vi "Autosort Get Sort Option.vi"(11 "Index":i32) -> (3 "Autosort Parameters":T1)   [LabVIEW 2016]
uses:
  Autosort Parameters.ctl
  Autosort Parameters Set.vi
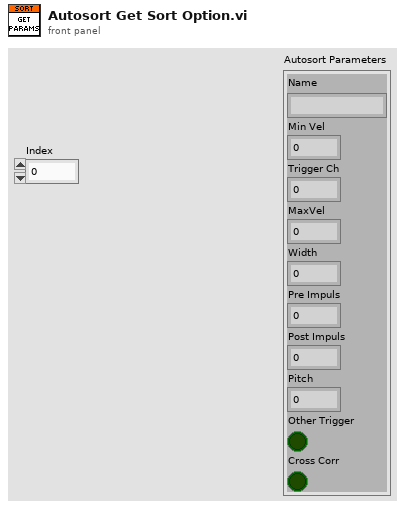
[diagram p1: front panel]
types:
  T1 = typedef "Autosort Parameters.ctl" = cluster{"Name":string, "Min Vel":dbl, "Trigger Ch":i32, "MaxVel":dbl, "Width":i32, "Pre Impuls":i32, "Post Impuls":i32, "Pitch":dbl, "Other Trigger":bool, "Cross Corr":bool}
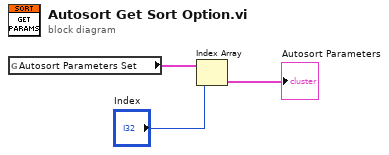
[diagram p0: block diagram]
diagram:
  n1 = global read "Autosort Parameters Set.vi" "Autosort Parameters Set"() -> (w3:T1[])
  n2 = Index Array(array=w3, index="Index") -> (element=→"Autosort Parameters":T1)
